vi "FP forebrain THINK.vi"(0 "GPS":cluster{"X pos":i32, "Y pos":i32, "Heading":dbl}={"X pos"=250, "Y pos"=250, "Heading"=0.0}, 1 "MDF index":i32, 2 "GPS?":bool=TRUE, 3 "MDF index docking":i32, 4 "Run?":bool=TRUE, 5 "error in":errorcluster, 6 "MDF in":T1(array[cluster])=[{"Type"=enum."Start", "X"=250, "Y"=250, "Speed"=0, "Behaviors"=enum."Open Water Transit"}, {"Type"=enum."Waypoint", "X"=400, "Y"=100, "Speed"=20, "Behaviors"=enum."P-Wall Follow"}, {"Type"=enum."Waypoint", "X"=250, "Y"=250, "Speed"=20, "Behaviors"=enum."Open Water Transit"}, {"Type"=enum."Waypoint", "X"=250, "Y"=400, "Speed"=20, "Behaviors"=enum."Open Water Transit"}, {"Type"=enum."Waypoint", "X"=100, "Y"=400, "Speed"=20, "Behaviors"=enum."Open Water Transit"}, {"Type"=enum."End", "X"=250, "Y"=250, "Speed"=0, "Behaviors"=enum."Open Water Transit"}], 7 "Tried Docking?":bool, 10 "Docking MDF In":T1(array[cluster])=[{"Type"=enum."Start", "X"=250, "Y"=250, "Speed"=0, "Behaviors"=enum."Open Water Transit"}, {"Type"=enum."Waypoint", "X"=400, "Y"=100, "Speed"=20, "Behaviors"=enum."P-Wall Follow"}, {"Type"=enum."Waypoint", "X"=250, "Y"=250, "Speed"=20, "Behaviors"=enum."Open Water Transit"}, {"Type"=enum."Waypoint", "X"=250, "Y"=400, "Speed"=20, "Behaviors"=enum."Open Water Transit"}, {"Type"=enum."Waypoint", "X"=100, "Y"=400, "Speed"=20, "Behaviors"=enum."Open Water Transit"}, {"Type"=enum."End", "X"=250, "Y"=250, "Speed"=0, "Behaviors"=enum."Open Water Transit"}], 15 "GPS Initial":cluster{"X pos":i32, "Y pos":i32, "Heading":dbl}={"X pos"=250, "Y pos"=250, "Heading"=0.0}) -> (11 "Docking MDF Out":T1(array[cluster])=[{"Type"=enum."Start", "X"=250, "Y"=250, "Speed"=0, "Behaviors"=enum."Open Water Transit"}, {"Type"=enum."Waypoint", "X"=400, "Y"=100, "Speed"=20, "Behaviors"=enum."P-Wall Follow"}, {"Type"=enum."Waypoint", "X"=250, "Y"=250, "Speed"=20, "Behaviors"=enum."Open Water Transit"}, {"Type"=enum."Waypoint", "X"=250, "Y"=400, "Speed"=20, "Behaviors"=enum."Open Water Transit"}, {"Type"=enum."Waypoint", "X"=100, "Y"=400, "Speed"=20, "Behaviors"=enum."Open Water Transit"}, {"Type"=enum."End", "X"=250, "Y"=250, "Speed"=0, "Behaviors"=enum."Open Water Transit"}], 12 "MDF Index out":i32, 13 "Complete?":bool=TRUE, 14 "Behaviors out":T2, 16 "local Steering\nangle":dbl, 17 "MDF Index out docking":i32, 18 "Tried Docking? Output":bool, 19 "error out":errorcluster)   [LabVIEW 2014]
panel:
  out "At Waypoint?":bool
  out "Forebrain Command":T3
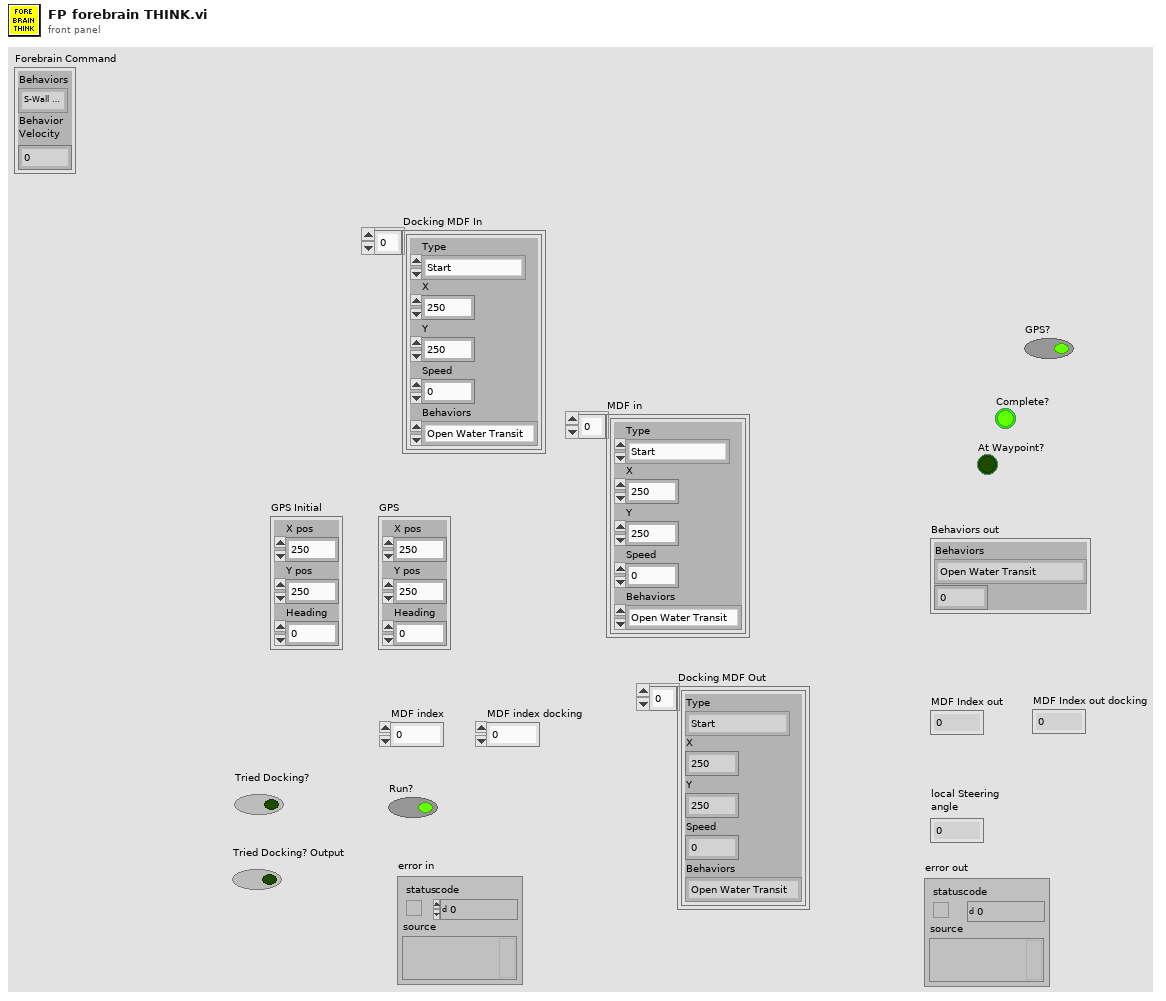
[diagram p1: front panel]
types:
  T1 = cluster{"Type":enum16{"Start", "Waypoint", "End"}, "X":i32, "Y":i32, "Speed":i32, "Behaviors":enum16{"Open Water Transit", "P-Wall Follow", "S-Wall Follow", "Dock"}}[]
  T2 = cluster{"Behaviors":enum16{"Open Water Transit", "P-Wall Follow", "S-Wall Follow", "Dock"}, dbl}
  T3 = cluster{"Behaviors":enum16{"S-Wall Follow", "P-Wall Follow", "Open Water Transit", "Get Unstuck"}, "Behavior\nVelocity":dbl}
  T4 = enum16{"Open Water Transit", "P-Wall Follow", "S-Wall Follow", "Dock"}
  T5 = cluster{"Type":enum16{"Start", "Waypoint", "End"}, "X":i32, "Y":i32, "Speed":i32, "Behaviors":enum16{"Open Water Transit", "P-Wall Follow", "S-Wall Follow", "Dock"}}
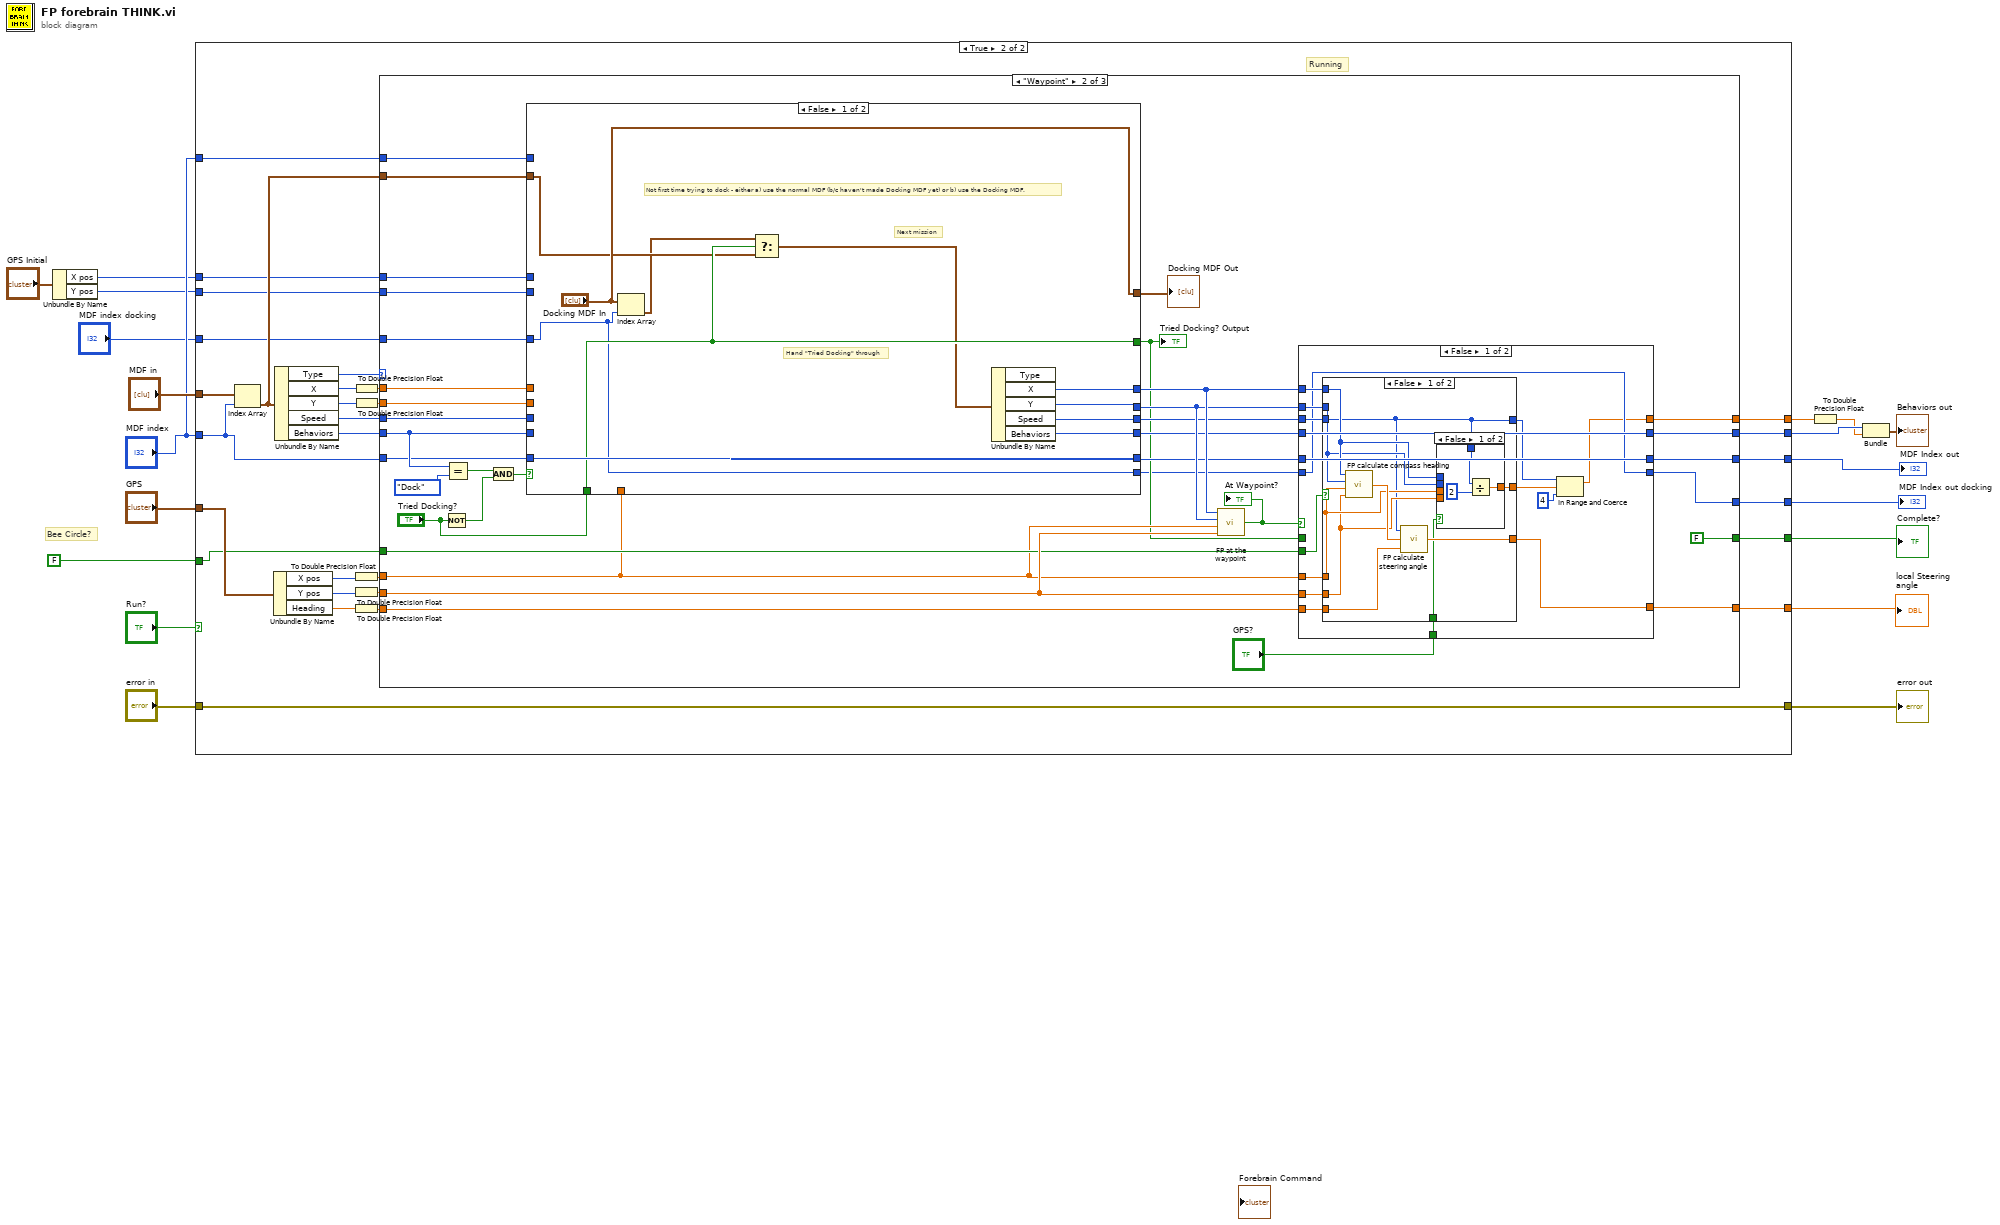
[diagram p0: block diagram]
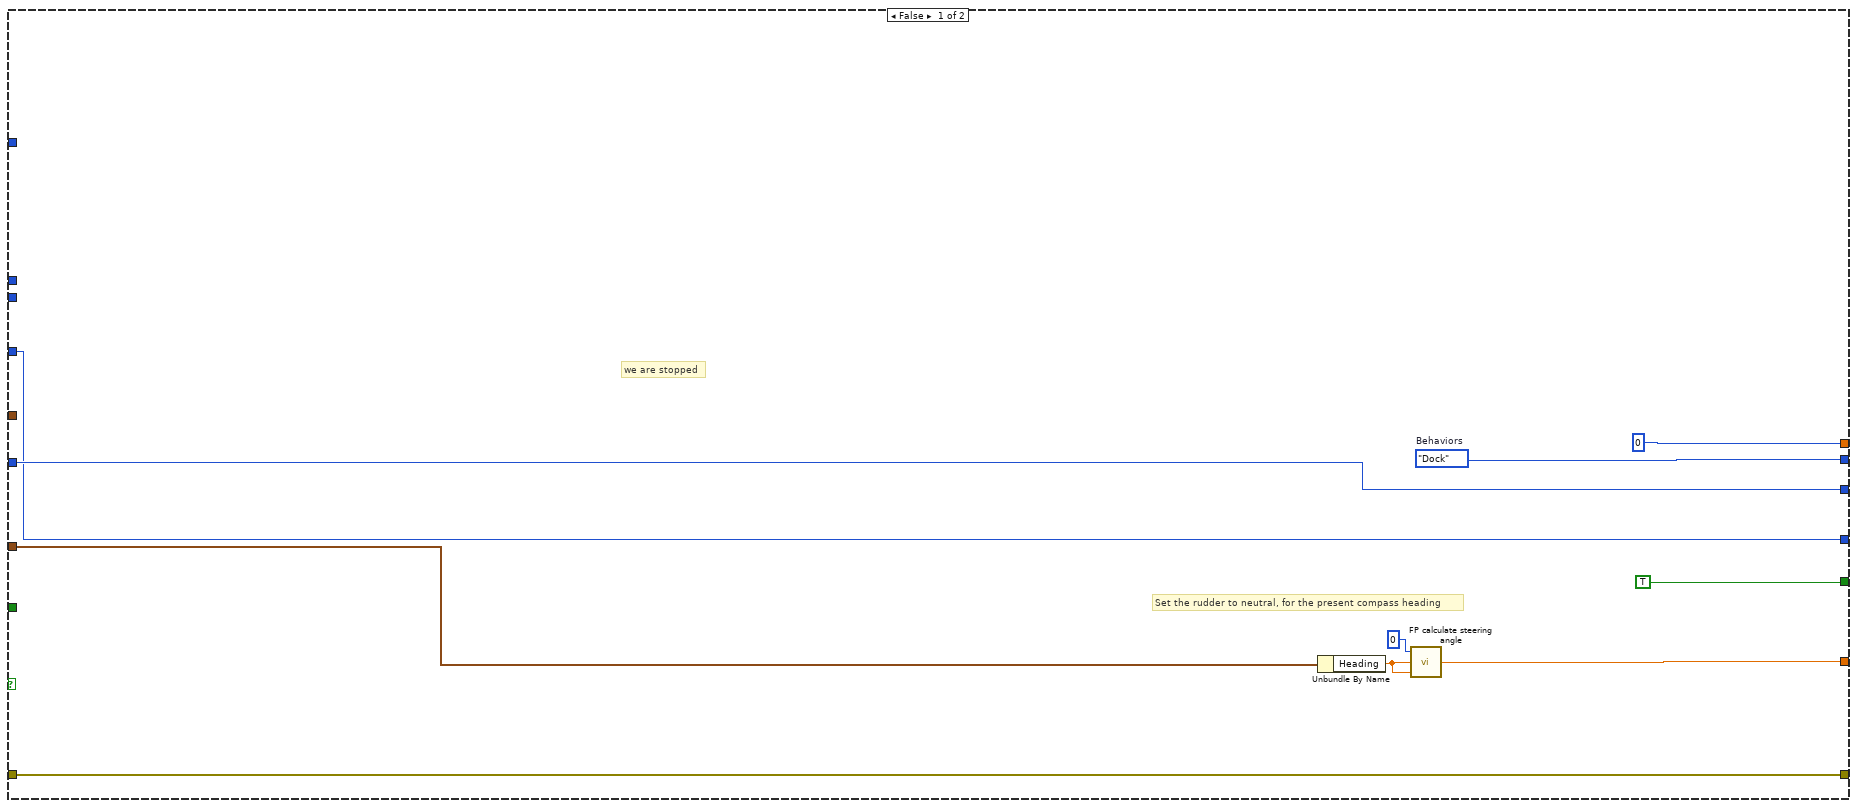
[diagram p2: hidden frame]
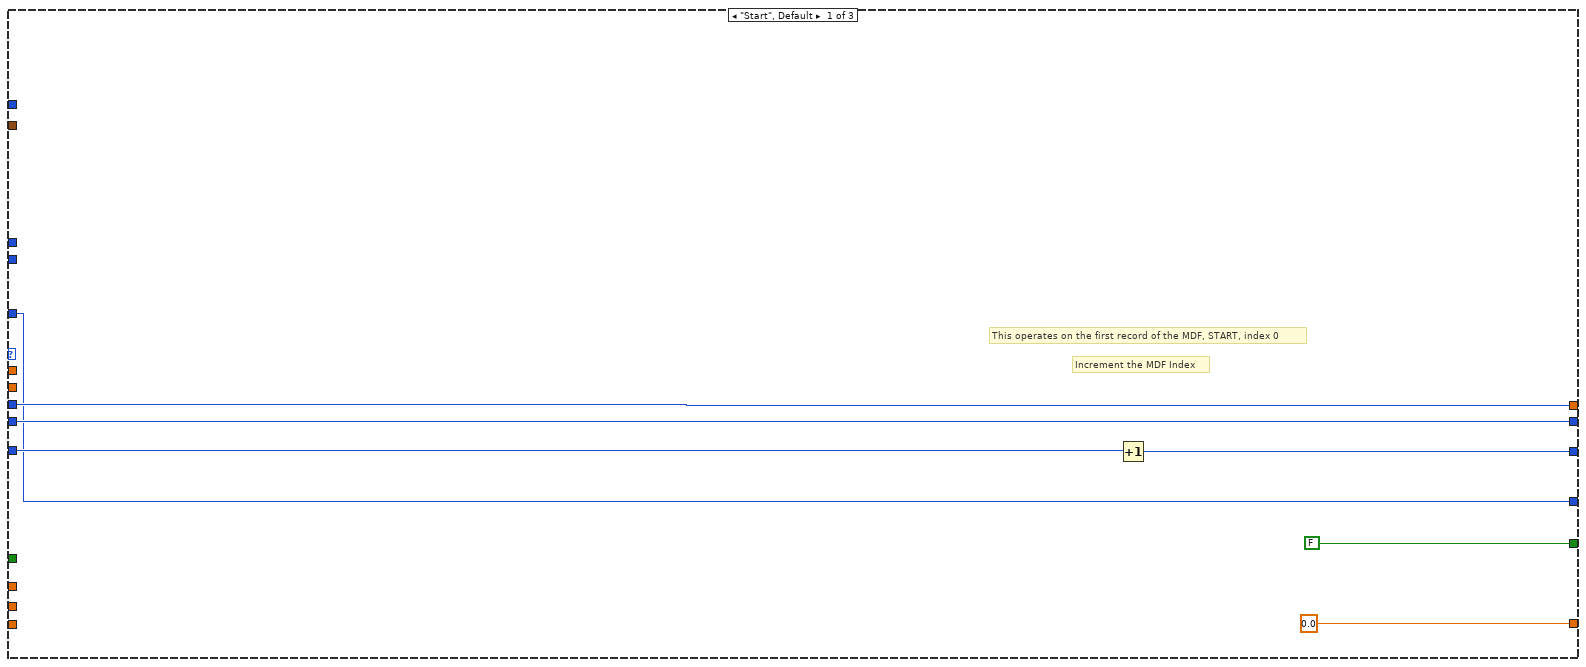
[diagram p3: hidden frame]
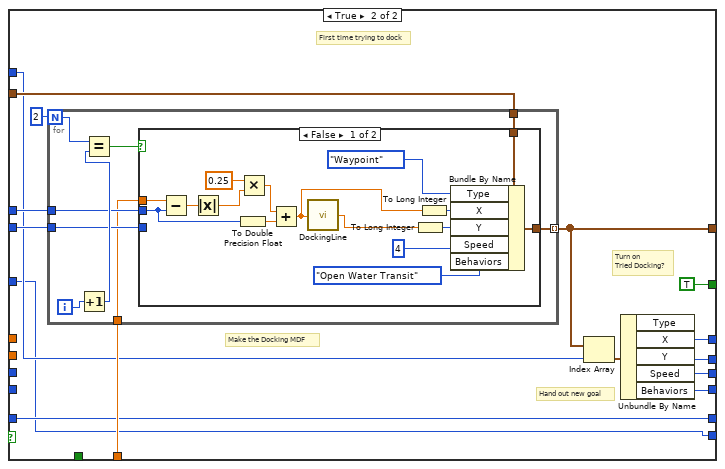
[diagram p4: hidden frame]
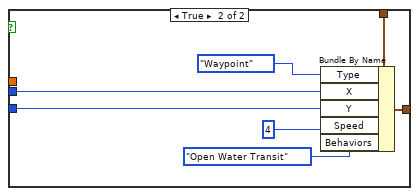
[diagram p5: hidden frame]
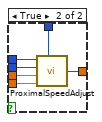
[diagram p6: hidden frame]
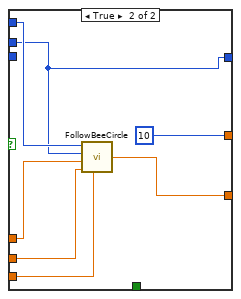
[diagram p7: hidden frame]
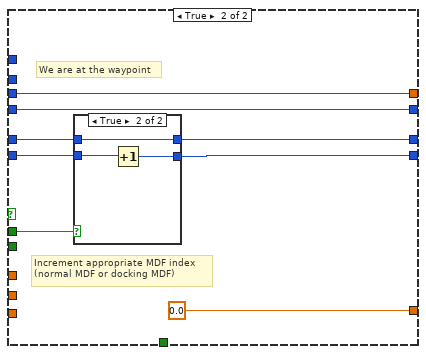
[diagram p8: hidden frame]
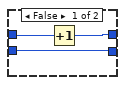
[diagram p9: hidden frame]
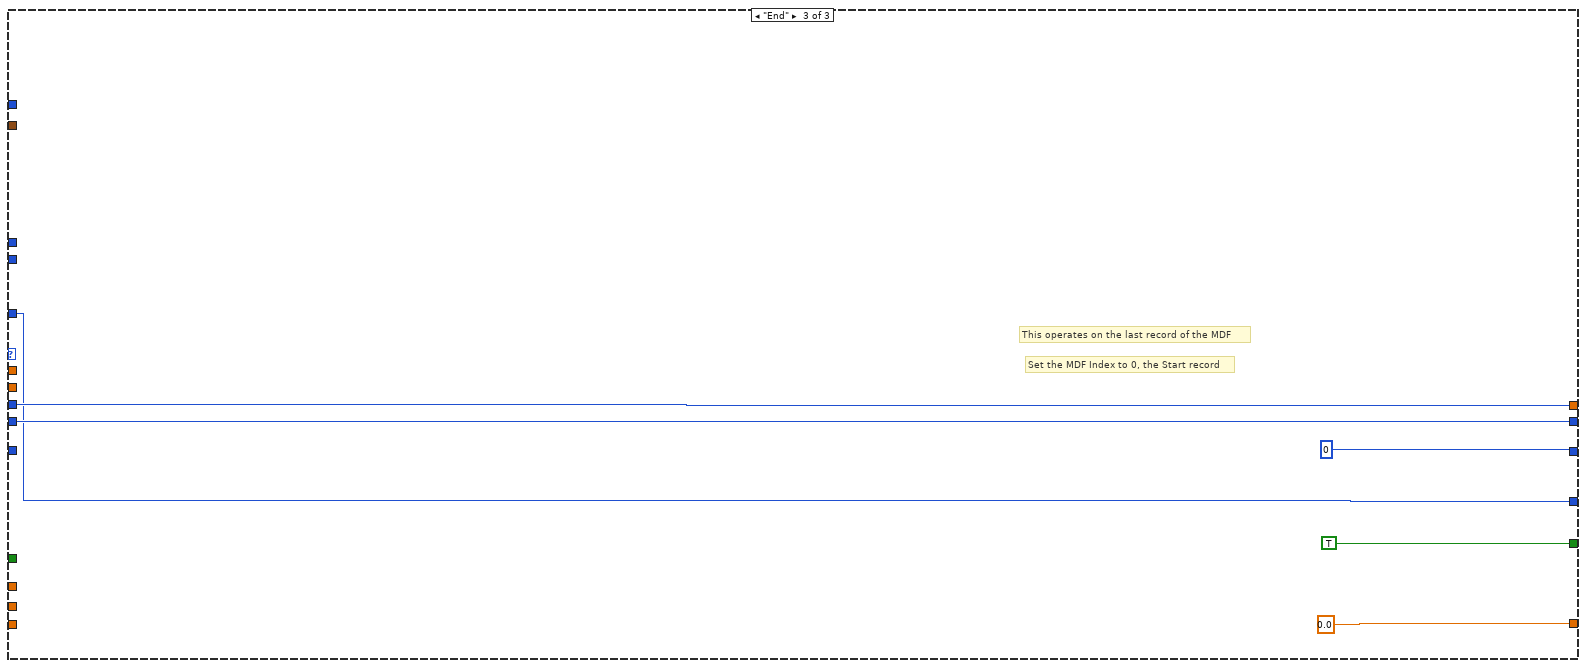
[diagram p10: hidden frame]
diagram:
  # "Bee Circle?"
  n1 = Unbundle By Name("GPS Initial") -> ("X pos"=w4:i32, "Y pos"=w3:i32)
  n2 = case shown="True" "Run?" {
    tunnel: "MDF in" -> [_ w58]
    tunnel: "MDF index" -> [w25 w44]
    tunnel: "error in" -> [w29 w56]
    tunnel: [w29 w56] -> w18
    tunnel: "GPS" -> [w28 w55]
    tunnel: [w25 w42] -> w15
    tunnel: [w26 w41] -> w14
    tunnel: [0 w39] -> w13
    tunnel: [w23 w38] -> w12
    tunnel: [TRUE w37] -> w9
    tunnel: FALSE -> [_ w36]
    tunnel: "MDF index" -> [_ w35]
    tunnel: w4 -> [_ w33]
    tunnel: w3 -> [_ w32]
    tunnel: "MDF index docking" -> [w20 w31]
    tunnel: [w20 w30] -> w1
    frame False {
      w23 = T4."Dock"  # Behaviors
      # "Set the rudder to neutral, for the present compass heading"
      # "we are stopped"
      n3 = Unbundle By Name(w28) -> ("Heading"=w27:dbl)
      n4 = call "FP calculate steering angle.vi"("Compass\nheading"=w27, "New heading"=w27, "Speed"=0) -> ("Local Steering Angle"=w26:dbl)
    }
    frame True {
      # "Running"
      n5 = Index Array(array=w58, index=w44) -> (element=w34:T5)
      n6 = Unbundle By Name(w55) -> ("X pos"=w52:i32, "Y pos"=w50:i32, "Heading"=w51:dbl)
      n7 = Unbundle By Name(w34) -> ("Type"=w57:enum16{"Start", "Waypoint", "End"}, "X"=w53:i32, "Y"=w54:i32, "Speed"=w40:i32, "Behaviors"=w43:T4)
      n8 = To Double Precision Float(number=w52) -> (double precision float=w47:dbl)
      n9 = To Double Precision Float(number=w50) -> (double precision float=w46:dbl)
      n10 = To Double Precision Float(number=w51) -> (double precision float=w45:dbl)
      n11 = To Double Precision Float(number=w53) -> (double precision float=w49:dbl)
      n12 = To Double Precision Float(number=w54) -> (double precision float=w48:dbl)
      n13 = case shown="\"Waypoint\"" w57 {
        tunnel: w49 -> [_ w90 _]
        tunnel: w48 -> [_ w88 _]
        tunnel: w47 -> [_ w76 _]
        tunnel: w46 -> [_ w96 _]
        tunnel: w45 -> [_ w95 _]
        tunnel: w44 -> [w63 w82 _]
        tunnel: [w62 w98 0] -> w42
        tunnel: w43 -> [w65 w84 w220]
        tunnel: [w65 w99 w220] -> w38
        tunnel: [0.0 w97 0.0] -> w41
        tunnel: w40 -> [w61 w86 w217]
        tunnel: [w61 w94 w217] -> w39
        tunnel: [FALSE FALSE TRUE] -> w37
        tunnel: w36 -> [_ w92 _]
        tunnel: w35 -> [_ w80 _]
        tunnel: w34 -> [_ w79 _]
        tunnel: w33 -> [_ w78 _]
        tunnel: w32 -> [_ w77 _]
        tunnel: w31 -> [w59 w70 w215]
        tunnel: [w59 w67 w215] -> w30
        frame "Start", Default {
          # "Increment the MDF Index"
          # "This operates on the first record of the MDF, START, index 0"
          n14 = Increment(x=w63) -> (x+1=w62:i32)
        }
        frame "Waypoint" {
          n15 = Not(x="Tried Docking?") -> (.not. x?=w72:bool)
          n16 = Equal?(x=w84, y=T4."Dock") -> (x = y?=w75:bool)
          n17 = And(x=w75, y=w72) -> (x .and. y?=w74:bool)
          n18 = case shown="False" w74 {
            tunnel: w90 -> [_ _]
            tunnel: [w107 w118] -> w89
            tunnel: w88 -> [_ _]
            tunnel: [w106 w117] -> w87
            tunnel: w86 -> [_ _]
            tunnel: [w105 w116] -> w85
            tunnel: w84 -> [_ _]
            tunnel: [w104 w115] -> w83
            tunnel: w82 -> [w111 w114]
            tunnel: [w111 w114] -> w81
            tunnel: w80 -> [_ w120]
            tunnel: w79 -> [w102 w126]
            tunnel: w78 -> [_ w124]
            tunnel: w77 -> [_ w123]
            tunnel: w76 -> [_ w122]
            tunnel: [w109 TRUE] -> w69
            tunnel: ["Docking MDF In" w113] -> w73
            tunnel: "Tried Docking?" -> [w109 _]
            tunnel: w70 -> [w103 w112]
            tunnel: [w103 w112] -> w68
            frame False {
              # "Hand \"Tried Docking\" through"
              # "Next mission"
              # "Not first time trying to dock - either a) use the normal MDF (b/c haven't made Docking MDF yet) or b) use the Docking MDF."
              n19 = Index Array(array="Docking MDF In", index=w103) -> (element=w101:T5)
              n20 = Select(t=w101, s=w109, f=w102) -> (s? t:f=w108:T5)
              n21 = Unbundle By Name(w108) -> ("X"=w107:i32, "Y"=w106:i32, "Speed"=w105:i32, "Behaviors"=w104:T4)  [unwired: 1 out]
            }
            frame True {
              # "Turn on\nTried Docking?"
              # "Hand out new goal"
              # "Make the Docking MDF"
              # "First time trying to dock"
              n22 = for {
                N: 2 -> [w134]
                tunnel: w126 -> [w135]
                tunnel: w124 -> [w130]
                tunnel: w123 -> [w129]
                tunnel: [w128] -> w113 mode=indexing
                tunnel: w122 -> [w127]
                i -> [w133]
                n23 = Increment(x=w133) -> (x+1=w132:i32)
                n24 = Equal?(x=w134, y=w132) -> (x = y?=w131:bool)
                n25 = case shown="False" w131 {
                  tunnel: w135 -> [w142 w158]
                  tunnel: w130 -> [w149 w154]
                  tunnel: w129 -> [_ w153]
                  tunnel: [w136 w152] -> w128
                  tunnel: w127 -> [w151 _]
                  frame False {
                    n26 = Subtract(x=w151, y=w149) -> (x-y=w150:dbl)
                    n27 = Absolute Value(x=w150) -> (abs(x)=w148:dbl)
                    n28 = To Double Precision Float(number=w149) -> (double precision float=w137:dbl)
                    n29 = Multiply(x=0.25, y=w148) -> (x*y=w146:dbl)
                    n30 = Add(x=w146, y=w137) -> (x+y=w140:dbl)
                    n31 = call "DockingLine.vi"("X"=w140) -> ("Y"=w141:dbl)
                    n32 = To Long Integer(number=w141) -> (32bit integer=w139:i32)
                    n33 = To Long Integer(number=w140) -> (32bit integer=w138:i32)
                    n34 = Bundle By Name(cluster=w142, "Type"=enum16{"Start", "Waypoint", "End"}."Waypoint", "X"=w138, "Y"=w139, "Speed"=4, "Behaviors"=T4."Open Water Transit") -> (w136:T5)
                  }
                  frame True {
                    n35 = Bundle By Name(cluster=w158, "Type"=enum16{"Start", "Waypoint", "End"}."Waypoint", "X"=w154, "Y"=w153, "Speed"=4, "Behaviors"=T4."Open Water Transit") -> (w152:T5)
                  }
                }
              }
              n36 = Index Array(array=w113, index=w120) -> (element=w119:T5)
              n37 = Unbundle By Name(w119) -> ("X"=w118:i32, "Y"=w117:i32, "Speed"=w116:i32, "Behaviors"=w115:T4)  [unwired: 1 out]
            }
          }
          "Tried Docking? Output" <- w69
          "Docking MDF Out" <- w73
          n38 = call "FP at the waypoint.vi"("Y location"=w96, "X location"=w76, "Yof waypoint"=w87, "X of waypoint"=w89) -> ("At Waypoint?"=w100:bool)
          "At Waypoint?" <- w100
          n39 = case shown="False" w100 {
            tunnel: w83 -> [w172 w208]
            tunnel: [w172 w208] -> w99
            tunnel: w81 -> [w173 w207]
            tunnel: [w173 w206] -> w98
            tunnel: [w164 0.0] -> w97
            tunnel: w76 -> [w168 _]
            tunnel: w96 -> [w167 _]
            tunnel: w95 -> [w174 _]
            tunnel: w89 -> [w170 _]
            tunnel: w87 -> [w169 _]
            tunnel: w85 -> [w171 w204]
            tunnel: [w159 w204] -> w94
            tunnel: w92 -> [w166 _]
            tunnel: w69 -> [_ w203]
            tunnel: w68 -> [w165 w202]
            tunnel: [w165 w201] -> w67
            tunnel: "GPS?" -> [w163 _]
            frame False {
              n40 = case shown="False" w166 {
                tunnel: w174 -> [w183 w197]
                tunnel: w171 -> [w175 _]
                tunnel: w170 -> [w182 w200]
                tunnel: w169 -> [w181 w194]
                tunnel: w168 -> [w180 w199]
                tunnel: w167 -> [w179 w198]
                tunnel: [w178 10 ("Desired Speed Out")] -> w162
                tunnel: [w177 w195] -> w164
                tunnel: w163 -> [w176 _]
                tunnel: [w175 w194] -> w160
                frame False {
                  n41 = call "FP calculate compass heading.vi"("Y Location"=w179, "X Location"=w180, "Waypoint Y"=w181, "Waypoint X"=w182) -> ("Heading"=w184:dbl)
                  n42 = call "FP calculate steering angle.vi"("Compass\nheading"=w183, "New heading"=w184, "Speed"=w175) -> ("Local Steering Angle"=w177:dbl)
                  n43 = case shown="False" w176 {
                    tunnel: w175 -> [w186 w193]
                    tunnel: w182 -> [_ w192]
                    tunnel: w181 -> [_ w191]
                    tunnel: w180 -> [_ w190]
                    tunnel: w179 -> [_ w189]
                    tunnel: [w187 w188] -> w178
                    frame False {
                      n44 = Divide(x=w186, y=2) -> (x/y=w187:dbl)
                    }
                    frame True {
                      n45 = call "ProximalSpeedAdjust.vi"("MDF X Position"=w192, "MDF Y Position"=w191, "GPS X Position"=w190, "GPS Y Position"=w189, "MDF Speed"=w193) -> ("Desired Speed Out"=w188:i32)
                    }
                  }
                }
                frame True {
                  n46 = call "FollowBeeCircle.vi"("Way Point X"=w200, "Way Point Y"=w194, "X Pos"=w199, "Y Pos"=w198, "Heading"=w197) -> ("Rudder Angle"=w195:dbl)
                }
              }
              n47 = In Range and Coerce(upper limit=w160, x=w162, lower limit=4) -> (coerced(x)=w159:dbl)  [unwired: 1 out]
            }
            frame True {
              # "We are at the waypoint"
              # "Increment appropriate MDF index\n(normal MDF or docking MDF)"
              n48 = case shown="True" w203 {
                tunnel: w207 -> [w210 w214]
                tunnel: [w209 w214] -> w206
                tunnel: w202 -> [w211 w213]
                tunnel: [w211 w212] -> w201
                frame False {
                  n49 = Increment(x=w210) -> (x+1=w209:i32)
                }
                frame True {
                  n50 = Increment(x=w213) -> (x+1=w212:i32)
                }
              }
            }
          }
        }
        frame "End" {
          # "Set the MDF Index to 0, the Start record"
          # "This operates on the last record of the MDF"
        }
      }
    }
  }
  "error out" <- w18
  "local Steering\nangle" <- w14
  "MDF Index out" <- w15
  "Complete?" <- w9
  "MDF Index out docking" <- w1
  n51 = To Double Precision Float(number=w13) -> (double precision float=w11:dbl)
  n52 = Bundle("Behaviors"=w12, w11) -> (→"Behaviors out":T2)  [unwired: 1 in]
